vi "Feeder Drop.vi"(8 "error in (no error)":errorcluster) -> (0 "error out":errorcluster)   [LabVIEW 2014]
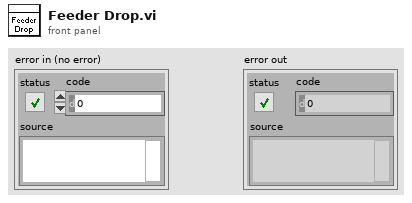
[diagram p1: front panel]
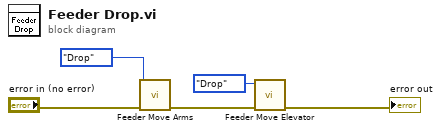
[diagram p0: block diagram]
diagram:
  n1 = call "Feeder Move Arms.vi"("error in (no error)"="error in (no error)", "Action"=enum16{"Drop", "Lift"}."Drop") -> ("error out"=w1:errorcluster)  [unwired: 9 in]
  n2 = call "Feeder Move Elevator.vi"("error in (no error)"=w1, "Action"=enum16{"Drop", "Lift"}."Drop") -> ("error out"=→"error out":errorcluster)  [unwired: 9 in]
